vi "PMBus Write Byte Ext.vi"(0 "DevType":i32, 1 "CommandCodeExt":u8, 2 "Data":u8, 5 "DevIndex":i32, 7 "PMBusIndex":i32, 9 "SlaveAddr":u8, 11 "error in (no error)":errorcluster, 12 "CommandCode":u8, 13 "PEC":u8) -> (4 "function return":i32, 15 "error out":errorcluster)   [LabVIEW 2012, in "ControlPMBus.lvlib"]
doc: "int WINAPI PMBus_WriteByteExt(int DevType,int DevIndex,int PMBusIndex,unsigned char SlaveAddr,unsigned char CommandCodeExt,unsigned char CommandCode,unsigned char Data,unsigned char PEC);"
uses:
  ControlPMBus.lvlib
  Ginkgo_Driver.dll
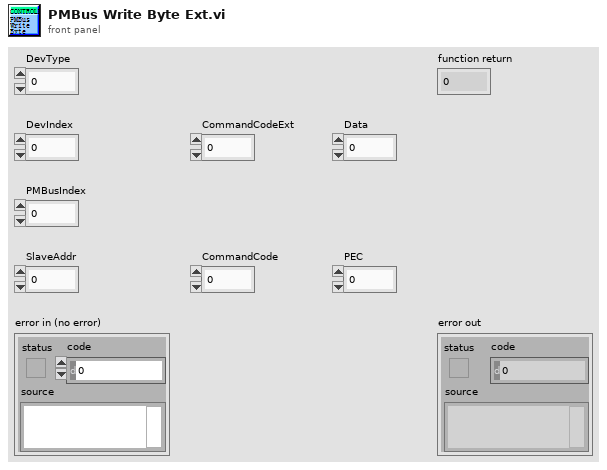
[diagram p1: front panel]
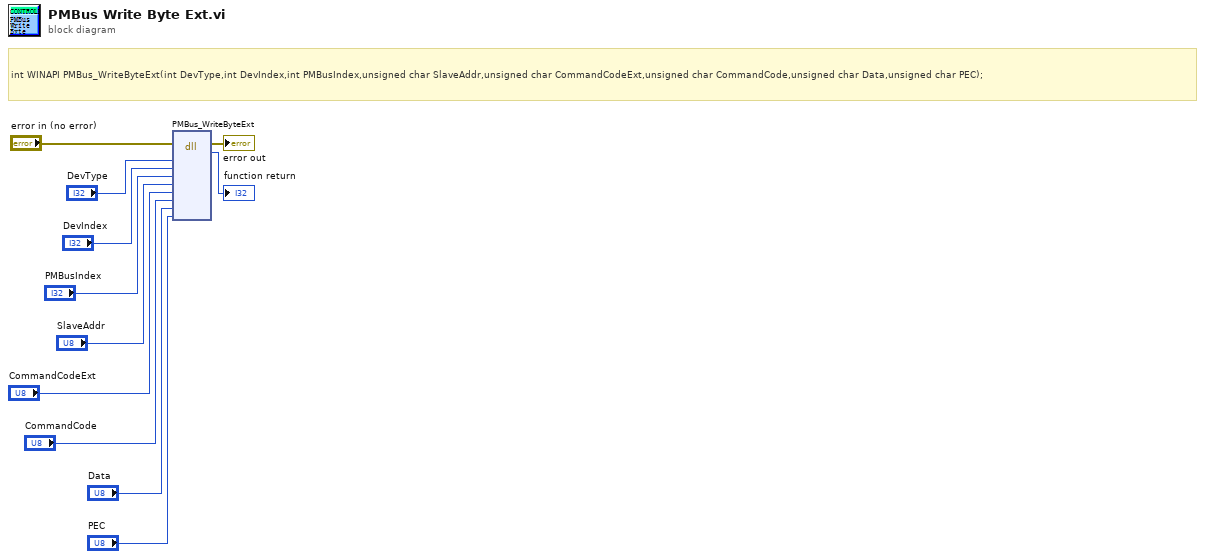
[diagram p0: block diagram]
diagram:
  # "int WINAPI PMBus_WriteByteExt(int DevType,int DevIndex,int PMBusIndex,unsigned char SlaveAddr,unsigned char CommandCodeExt,unsigned char CommandCode,unsigned char Data,unsigned char PEC);"
  n1 = dll-call lib="E:/Project/vt_ginkgo/truck/Ginkgo Driver/vs2010/Ginkgo_USB-I2C_API_v2.0.3.0/lib/labview_64bit/ControlPMBus/Ginkgo_Driver.*" fn="PMBus_WriteByteExt"(error in="error in (no error)", "DevType"="DevType", "DevIndex"="DevIndex", "PMBusIndex"="PMBusIndex", "SlaveAddr"="SlaveAddr", "CommandCodeExt"="CommandCodeExt", "CommandCode"="CommandCode", "Data"="Data", "PEC"="PEC") -> (error out=→"error out":errorcluster, →"function return":i32)  [unwired: 10 in, 1 out]
